vi "get channels.vi"(11 "module configuration in":refnum<class "asynchronous execution module configuration.lvclass">) -> (2 "channels":refnum<class "TBM channel.lvclass">[](array[class]), 3 "module configuration out":refnum<class "asynchronous execution module configuration.lvclass">)   [LabVIEW 2013, in "asynchronous execution module configuration.lvclass"]
uses:
  asynchronous execution module configuration.lvclass
  <vilib>/NI/Tag Bus Module Framework/channel/TBM channel.lvclass
  asynchronous execution module configuration.lvclass/asynchronous execution module configuration.ctl
  <vilib>/NI/Tag Bus Module Framework/module configuration/TBM module configuration.lvclass
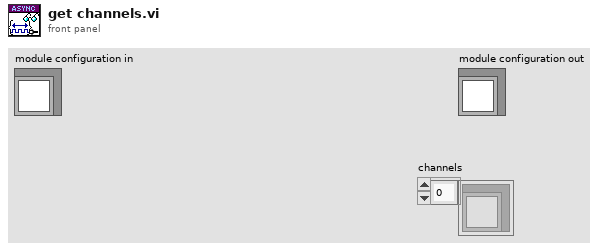
[diagram p1: front panel]
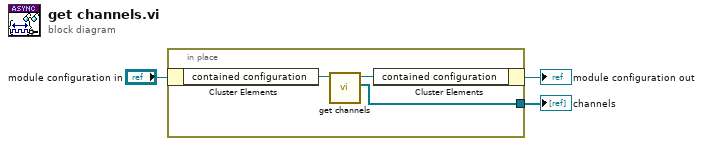
[diagram p0: block diagram]
diagram:
  n1 = in-place {
    in-place-border: [w4] -> w3
    n2 = in-place-cluster #1("module configuration in") -> ("contained configuration"=w6:refnum<class "TBM module configuration.lvclass">)
    n3 = call-dynamic "get channels.vi"("module configuration in"=w6) -> ("channels"=w4:refnum<class "TBM channel.lvclass">[], "module configuration out"=w5:refnum<class "TBM module configuration.lvclass">)  [unwired: 9 in]
    n4 = in-place-cluster #1("contained configuration"=w5) -> (→"module configuration out":refnum<class "asynchronous execution module configuration.lvclass">)
  }
  "channels" <- w3
